vi "ge_ClearBoneyard.vi"(8 "error in":errorcluster, 11 "FP Ctrl":T1) -> (0 "error out":errorcluster)   [LabVIEW 2012]
uses:
  Custom Ctrls/ge_FPCtrlRefLabel.ctl
  <vilib>/Utility/miscctls.llb/LVPositionTypeDef.ctl
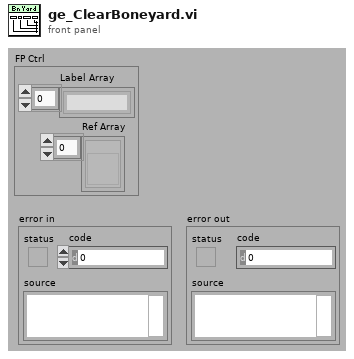
[diagram p1: front panel]
types:
  T1 = typedef "ge_FPCtrlRefLabel.ctl" = cluster{"Label Array":string[], "Ref Array":refnum<vi>[]}
  T2 = typedef "LVPositionTypeDef.ctl" = cluster{"Left":i32, "Top":i32}
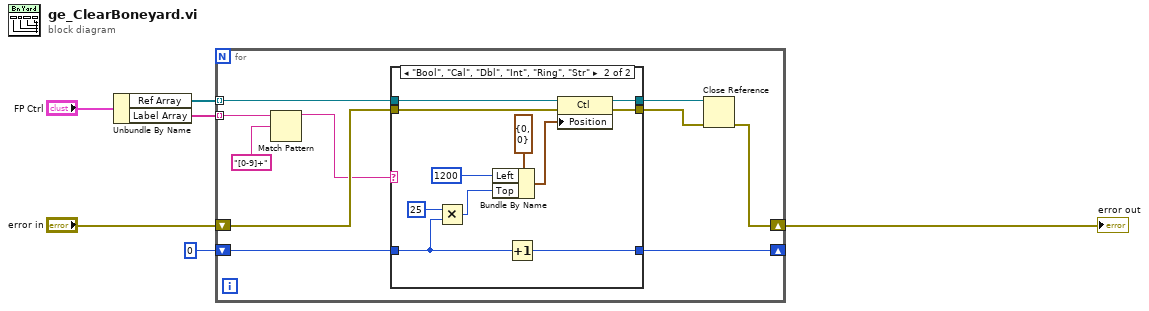
[diagram p0: block diagram]
diagram:
  n1 = Unbundle By Name("FP Ctrl") -> ("Ref Array"=w3:refnum<vi>[], "Label Array"=w2:string[])
  n2 = for {
    shift-right: [w14] -> w5
    shift-left: "error in" -> [w13]
    tunnel: w3 -> [w12] mode=indexing
    tunnel: w2 -> [w10] mode=indexing
    shift-right: [w7] -> _
    shift-left: 0 -> [w8]
    n3 = Match Pattern(string=w10, regular expression="[0-9]+") -> (before substring=w9:string)  [unwired: 1 in, 3 out]
    n4 = case shown="\"Bool\", \"Cal\", \"Dbl\", \"Int\", \"Ring\", \"Str\"" w9 {
      tunnel: w8 -> [w17 w21]
      tunnel: [w19 w25] -> w16
      tunnel: [w18 w24] -> w15
      tunnel: w13 -> [w18 w23]
      tunnel: w12 -> [w19 w22]
      tunnel: [w17 w20] -> w7
      frame Default {
      }
      frame "Bool", "Cal", "Dbl", "Int", "Ring", "Str" {
        n5 = Multiply(x=25, y=w21) -> (x*y=w26:i32)
        n6 = Bundle By Name(cluster=T2 {"Left"=0, "Top"=0} ("Position"), "Left"=1200, "Top"=w26) -> (w29:T2)
        n7 = Increment(x=w21) -> (x+1=w20:i32)
        n8 = property class="Ctl"(reference=w22, error in=w23, "Position"=w29) -> (reference out=w25:refnum<vi>, error out=w24:errorcluster)
      }
    }
    n9 = Close Reference(reference=w16, error in (no error)=w15) -> (error out=w14:errorcluster)
  }
  "error out" <- w5
